vi "AlliGator Get-Set Background Dataset Options.vi"(8 "error in (no error)":errorcluster, 9 "Background Dataset":bool, 10 "Image Loading Options":T4={"Pixel Well Capacity"=0, "Pile-up Correction"=FALSE, "Gate Step"=0, "Image Smoothing Options"={"Use Image Smoothing"=FALSE, "Kernel Type"=enum."Bilinear", "Bin"=1, "Algorithm"=enum."Rapid"}, "Gates to Skip"={"Start"=0, "End"=0}, "File Background Subtraction"=FALSE, "Background File Path"=path "", "Image Binning Options"={"Use Image Binning"=FALSE, "X Bin"=1, "Y Bin"=1}, "# Gates"=0, "Gates to Keep"={"First"=0, "Last"=0}, "Define Gates to"=FALSE, "Hot Pixel Removal"={"Remove Screamers"=FALSE, "Delta"=0.0, "Equalize Histogram"=FALSE, "Percentile"=0.0, "Hot Pixel Mask Image"=path "", "Use Hot Pixel Mask"=FALSE}, "Dataset Scaling Factor"=0.0, "Image Pre-processing Steps"=[]} {"Hot Pixel Removal"."Percentile" min=0 max=100; "Image Binning Options"."Y Bin" min=1; "Image Binning Options"."X Bin" min=1; "Image Smoothing Options"."Bin" min=1}, 11 "FLI Data File Information":T1) -> (0 "error out":errorcluster, 1 "Load Dataset?":bool)   [LabVIEW 2021, in "AlliGator Files.lvlib"]
doc: "Compares file parameters and loading options to previously stored one (if this is a background file).\nIf no change, return FALSE to skip data loading, since we already have this data in memory."
uses:
  AlliGator Files.lvlib
  AlliGator Image Loading Options.ctl
  AlliGator Image Smoothing Options.ctl
  Arrays/Kernel Type.ctl
  Arrays/Smoothing Algorithm.ctl
  AlliGator Gates to Skip.ctl
  AlliGator Image Binning Options.ctl
  AlliGator Gates to Keep.ctl
  SwissSPAD/SwissSPAD Live_Image Display Options.ctl
  AlliGator Image Pre-processing Step.ctl
  AlliGator FLI Data File Information.ctl
  Phasor/Phasor Fluorescence Lifetime Parameters v3.ctl
  AlliGator FLI Dataset Type.ctl
  342f137a-404f-49a2-b0fe-3d5e90135ae4.vi
  eb7c5d63-399e-479a-82b4-bf470f0d7762.vi
  Arrays/Arrays.lvlib
  AlliGator Settings.lvlib
  AlliGator Decay Analysis.lvlib
  AlliGator Source Image.lvlib
  AlliGator HDF5.lvlib
  SwissSPAD/SwissSPAD Live.lvlib
  Phasor/Phasor.lvlib
panel:
  # "see the AlliGator License on the block diagram (Ctrl+E or Window:Show Block Diagram)"
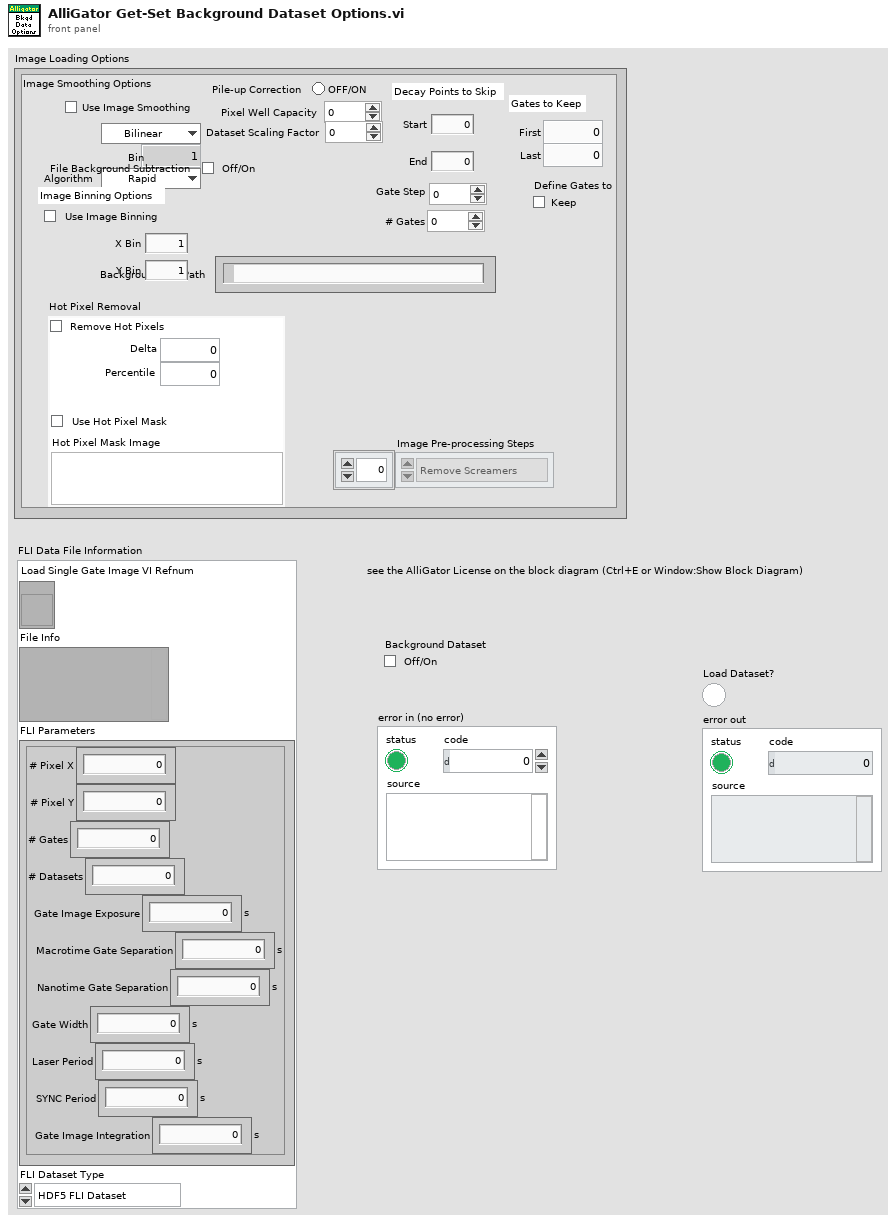
[diagram p1: front panel]
types:
  T1 = typedef "AlliGator HDF5.lvlib/AlliGator FLI Data File Information.ctl" = cluster{"Load Single Gate Image VI Refnum":refnum<vi>, "File Info":variant, "FLI Parameters":T2, "FLI Dataset Type":T3}
  T2 = typedef "Phasor.lvlib/Phasor Fluorescence Lifetime Parameters v3.ctl" = cluster{"# Pixel X":i32, "# Pixel Y":i32, "# Gates":i32, "# Datasets":i32, "Gate Image Exposure":dbl[unit], "Macrotime Gate Separation":dbl[unit], "Nanotime Gate Separation":dbl[unit], "Gate Width":dbl[unit], "Laser Period":dbl[unit], "SYNC Period":dbl[unit], "Gate Image Integration":dbl[unit]}
  T3 = typedef "AlliGator Files.lvlib/AlliGator FLI Dataset Type.ctl" = enum16{"HDF5 FLI Dataset", "Gate Image Folder", ".sdt FLI Dataset (Becker & Hickl)", ".ptu FLI Dataset (PicoQuant)", "SS1 FLI Dataset", "SS2 FLI Dataset", "I/m/phi Dataset", ".bin FLI Dataset (PicoQuant Binned)", ".bin FLI Dataset (Piccolo Binned)"}
  T4 = typedef "AlliGator Source Image.lvlib/AlliGator Image Loading Options.ctl" = cluster{"Pixel Well Capacity":u32, "Pile-up Correction":bool, "Gate Step":i32, "Image Smoothing Options":T5, "Gates to Skip":T8, "File Background Subtraction":bool, "Background File Path":path, "Image Binning Options":T9, "# Gates":u32, "Gates to Keep":T10, "Define Gates to":bool, "Hot Pixel Removal":T11, "Dataset Scaling Factor":dbl, "Image Pre-processing Steps":T12[]}
  T5 = typedef "AlliGator Settings.lvlib/AlliGator Image Smoothing Options.ctl" = cluster{"Use Image Smoothing":bool, "Kernel Type":T6, "Bin":i32, "Algorithm":T7}
  T6 = typedef "Arrays.lvlib/Kernel Type.ctl" = enum16{"Uniform", "Bilinear", "Gaussian"}
  T7 = typedef "Arrays.lvlib/Smoothing Algorithm.ctl" = enum16{"Rapid", "Thorough"}
  T8 = typedef "AlliGator Decay Analysis.lvlib/AlliGator Gates to Skip.ctl" = cluster{"Start":u32, "End":u32}
  T9 = typedef "AlliGator Source Image.lvlib/AlliGator Image Binning Options.ctl" = cluster{"Use Image Binning":bool, "X Bin":i32, "Y Bin":i32}
  T10 = typedef "AlliGator Settings.lvlib/AlliGator Gates to Keep.ctl" = cluster{"First":u32, "Last":u32}
  T11 = typedef "SwissSPAD Live.lvlib/SwissSPAD Live_Image Display Options.ctl" = cluster{"Remove Screamers":bool, "Delta":sgl, "Equalize Histogram":bool, "Percentile":sgl, "Hot Pixel Mask Image":path, "Use Hot Pixel Mask":bool}
  T12 = typedef "AlliGator Files.lvlib/AlliGator Image Pre-processing Step.ctl" = enum16{"Remove Screamers", "Pile-up Correction", "Binning", "Smoothing", "Rescaling", "Dead Left Column Correction"}
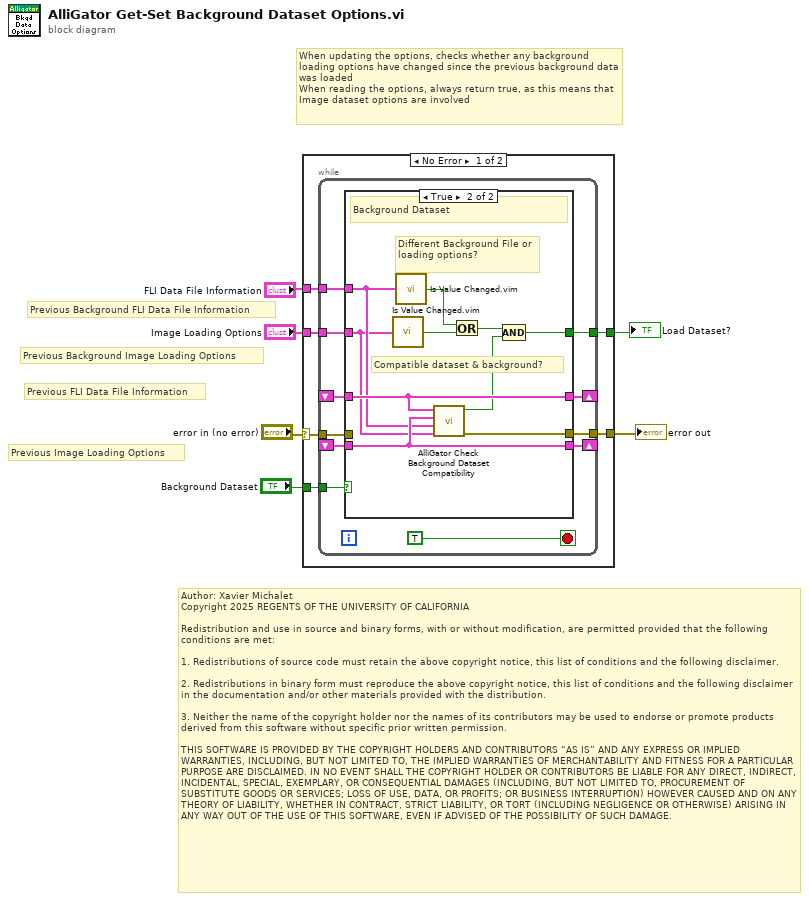
[diagram p0: block diagram]
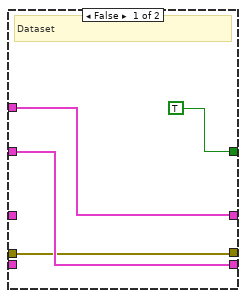
[diagram p2: hidden frame]
diagram:
  # "Author: Xavier Michalet\nCopyright 2025 REGENTS OF THE UNIVERSITY OF CALIFORNIA\n\nRedistribution and use in source and binary forms, with or without modification, are permitted provided that the following conditions are met:\n\n1. Redistributions of source code must retain the above copyright notice, this list of conditions and the following disclaimer.\n\n2. Redistributions in binary form must reproduce the above copyright notice, this list of conditions and the following disclaimer in the documentation and/or other materials provided with the distribution.\n\n3. Neither the name of the copyright holder nor the names of its contributors may be used to endorse or promote products derived from this software without specific prior written permission.\n\nTHIS SOFTWARE IS PROVIDED BY THE COPYRIGHT HOLDERS AND CONTRIBUTORS “AS IS” AND ANY EXPRESS OR IMPLIED WARRANTIES, INCLUDING, BUT NOT LIMITED TO, THE IMPLIED WARRANTIES OF MERCHANTABILITY AND FITNESS FOR A PARTICULAR PURPOSE ARE DISCLAIMED. IN NO EVENT SHALL THE COPYRIGHT HOLDER OR CONTRIBUTORS BE LIABLE FOR ANY DIRECT, INDIRECT, INCIDENTAL, SPECIAL, EXEMPLARY, OR CONSEQUENTIAL DAMAGES (INCLUDING, BUT NOT LIMITED TO, PROCUREMENT OF SUBSTITUTE GOODS OR SERVICES; LOSS OF USE, DATA, OR PROFITS; OR BUSINESS INTERRUPTION) HOWEVER CAUSED AND ON ANY THEORY OF LIABILITY, WHETHER IN CONTRACT, STRICT LIABILITY, OR TORT (INCLUDING NEGLIGENCE OR OTHERWISE) ARISING IN ANY WAY OUT OF THE USE OF THIS SOFTWARE, EVEN IF ADVISED OF THE POSSIBILITY OF SUCH DAMAGE."
  # "Previous Image Loading Options"
  # "Previous FLI Data File Information"
  # "Previous Background Image Loading Options"
  # "Previous Background FLI Data File Information"
  # "When updating the options, checks whether any background loading options have changed since the previous background data was loaded\nWhen reading the options, always return true, as this means that Image dataset options are involved"
  n1 = case shown="No Error" "error in (no error)" {
    selector: "error in (no error)" -> [w7 w38]
    tunnel: "Background Dataset" -> [w12 _]
    tunnel: [w11 _] -> w6
    tunnel: "FLI Data File Information" -> [w10 _]
    tunnel: "Image Loading Options" -> [w9 _]
    tunnel: [w8 w38] -> w1
    frame No Error {
      n2 = while {
        tunnel: w12 -> [w22]
        tunnel: w10 -> [w21]
        tunnel: [w20] -> w11
        tunnel: w9 -> [w19]
        shift-right: [w17] -> _
        shift-left: _ -> [w16]
        shift-right: [w18] -> _
        shift-left: _ -> [w15]
        tunnel: [w14] -> w8
        tunnel: w7 -> [w13]
        stop <- TRUE stop-if-true
        n3 = case shown="True" w22 {
          tunnel: w21 -> [w26 w31]
          tunnel: [TRUE w34] -> w20
          tunnel: w19 -> [w25 w29]
          tunnel: [w26 w36] -> w17
          tunnel: [w25 w35] -> w18
          tunnel: w16 -> [_ w36]
          tunnel: w15 -> [_ w35]
          tunnel: [w24 w32] -> w14
          tunnel: w13 -> [w24 _]
          frame False {
            # "Dataset"
          }
          frame True {
            # "Compatible dataset & background?"
            # "Different Background File or loading options?"
            # "Background Dataset"
            n4 = call "Is Value Changed.vim"("value"=w29) -> ("changed or first call?"=w28:bool)
            n5 = call "Is Value Changed.vim"("value"=w31) -> ("changed or first call?"=w30:bool)
            n6 = call "AlliGator Check Background Dataset Compatibility.vi"("Background Image Loading Options"=w29, "Background FLI Data File Information"=w31, "Dataset Image Loading Options"=w35, "Dataset FLI Data File Information"=w36) -> ("Error Out"=w32:errorcluster, "Compatible Background Dataset?"=w33:bool)  [unwired: 6 in]
            n7 = Or(x=w30, y=w28) -> (x .or. y?=w37:bool)
            n8 = Compound Arithmetic op=AND(w37, w33) -> (w34:bool)
          }
        }
      }
    }
    frame Error {
    }
  }
  "error out" <- w1
  "Load Dataset?" <- w6
